vi "CycleRemoveItem.vi"(11 "TreeControl输入":refnum<vi>) -> (0 "删除行索引":i32, 1 "删除成功":bool, 3 "TreeControl输出":refnum<vi>)   [LabVIEW 2020, in "Curve Editor.lvlib"]
uses:
  Curve Editor.lvlib
panel:
  # "删除树形中选中的子标识，并返回删了掉的标识的行索引"
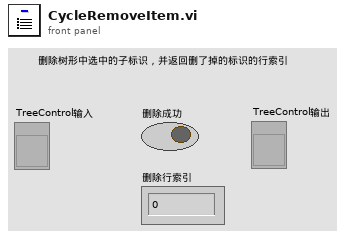
[diagram p1: front panel]
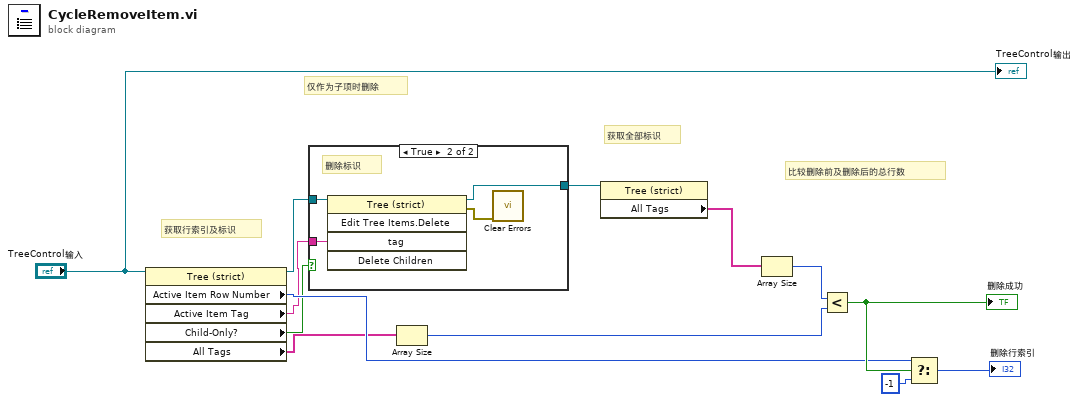
[diagram p0: block diagram]
diagram:
  # "比较删除前及删除后的总行数"
  # "获取全部标识"
  # "仅作为子项时删除"
  # "获取行索引及标识"
  n1 = property class="Tree (strict)"(reference="TreeControl输入") -> (reference out=w4:refnum<vi>, "Active Item Row Number"=w7:i32, "Active Item Tag"=w5:string, "Child-Only?"=w6:bool, "All Tags"=w3:string[])  [unwired: 1 in, 1 out]
  n2 = case shown="True" w6 {
    tunnel: w4 -> [w14 w18]
    tunnel: w5 -> [_ w17]
    tunnel: [w14 w16] -> w10
    frame False {
    }
    frame True {
      # "删除标识"
      n3 = invoke class="Tree (strict)" method="Edit Tree Items.Delete"(reference=w18, "tag"=w17) -> (reference out=w16:refnum<vi>, error out=w15:errorcluster)  [unwired: 3 in, 3 out]
      n4 = call <vilib>:"Clear Errors.vi"("error in (no error)"=w15) -> ()  [unwired: 5 in, 2 out]
    }
  }
  n5 = Array Size(array=w3) -> (size(s)=w2:i32)
  n6 = property class="Tree (strict)"(reference=w10) -> ("All Tags"=w11:string[])  [unwired: 1 in, 2 out]
  n7 = Array Size(array=w11) -> (size(s)=w12:i32)
  n8 = Less?(x=w12, y=w2) -> (x < y?=w13:bool)
  "删除成功" <- w13
  n9 = Select(t=w7, s=w13, f=-1) -> (s? t:f=→"删除行索引":i32)
  "TreeControl输出" <- "TreeControl输入"
